vi "Basic_Control_SubVI.vi"(0 "Numeric 2":dbl, 1 "Numeric":dbl, 2 "Numeric 10":dbl, 3 "Numeric 8":dbl, 4 "Numeric 9":dbl, 5 "Numeric 7":dbl, 6 "Numeric 6":dbl, 8 "Numeric 3":dbl, 9 "Tolerance":dbl, 10 "Numeric 4":dbl, 11 "duty cycle (periods) 5":fxp<+,32,0>, 12 "Numeric 5":dbl) -> (16 "Colision?":bool, 18 "duty cycle (periods) 4":fxp<+,32,0>, 19 "Mod1/Drive Direction 2":enum8{"Clockwise", "Counterclockwise"}(ring), 20 "Mod1/Drive Direction 6":enum8{"Clockwise", "Counterclockwise"}(ring), 21 "duty cycle (periods) 3":fxp<+,32,0>, 22 "Mod1/Drive Direction 5":enum8{"Clockwise", "Counterclockwise"}(ring), 23 "duty cycle (periods) 2":fxp<+,32,0>, 24 "Mod1/Drive Direction 4":enum8{"Clockwise", "Counterclockwise"}(ring), 25 "Mod1/Drive Direction 3":enum8{"Clockwise", "Counterclockwise"}(ring), 26 "duty cycle (periods)":fxp<+,32,0>)   [LabVIEW 2014]
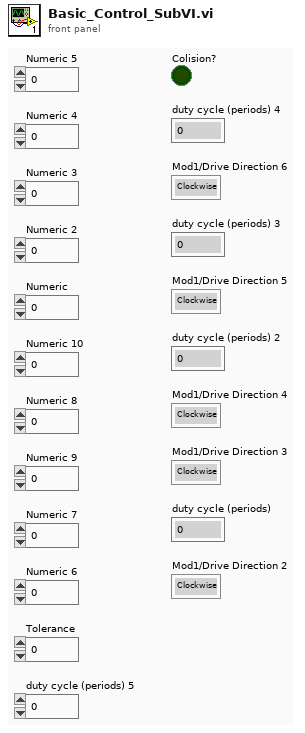
[diagram p1: front panel]
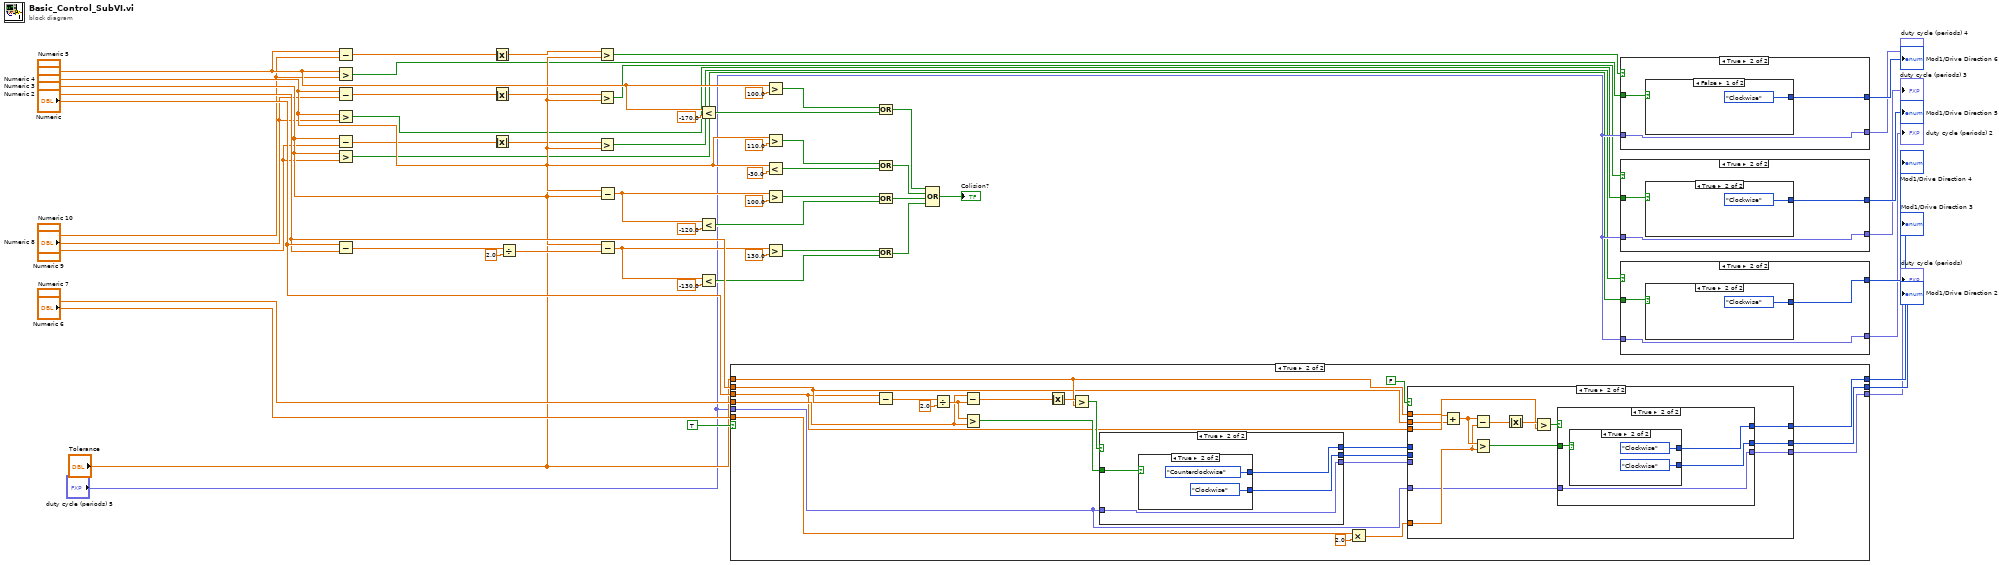
[diagram p0: block diagram]
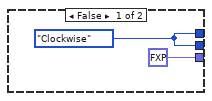
[diagram p2: hidden frame]
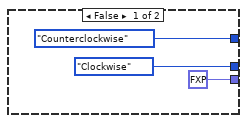
[diagram p4: hidden frame]
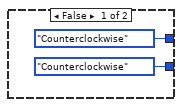
[diagram p5: hidden frame]
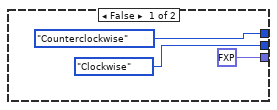
[diagram p6: hidden frame]
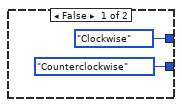
[diagram p7: hidden frame]
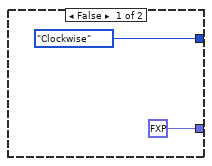
[diagram p8: hidden frame]
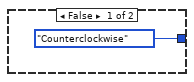
[diagram p9: hidden frame]
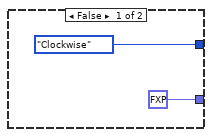
[diagram p10: hidden frame]
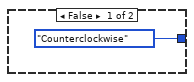
[diagram p11: hidden frame]
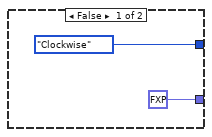
[diagram p12: hidden frame]
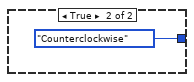
[diagram p13: hidden frame]
diagram:
  n1 = Subtract(x="Numeric 5", y="Numeric 10") -> (x-y=w5:dbl)
  n2 = Greater?(x="Numeric 5", y="Numeric 10") -> (0:w1:bool)
  n3 = Subtract(x="Numeric 4", y="Numeric 8") -> (x-y=w12:dbl)
  n4 = Greater?(x="Numeric 4", y="Numeric 8") -> (0:w2:bool)
  n5 = Subtract(x="Numeric 3", y="Numeric 9") -> (x-y=w9:dbl)
  n6 = Greater?(x="Numeric 3", y="Numeric 9") -> (0:w3:bool)
  n7 = Subtract(x="Numeric", y="Numeric 2") -> (x-y=w49:dbl)
  n8 = Absolute Value(x=w5) -> (abs(x)=w6:dbl)
  n9 = Absolute Value(x=w12) -> (abs(x)=w13:dbl)
  n10 = Absolute Value(x=w9) -> (abs(x)=w10:dbl)
  n11 = Divide(x=w49, y=2.0) -> (x/y=w50:dbl)
  n12 = Greater?(x=w6, y="Tolerance") -> (0:w7:bool)
  n13 = Greater?(x=w13, y="Tolerance") -> (0:w14:bool)
  n14 = Greater?(x=w10, y="Tolerance") -> (0:w15:bool)
  n15 = Subtract(x="Numeric 4", y="Numeric 3") -> (x-y=w29:dbl)
  n16 = Subtract(x="Numeric 3", y=w50) -> (x-y=w34:dbl)
  n17 = Less?(x="Numeric 5", y=-170.0) -> (x < y?=w22:bool)
  n18 = Less?(x=w29, y=-120.0) -> (x < y?=w33:bool)
  n19 = Less?(x=w34, y=-130.0) -> (x < y?=w38:bool)
  n20 = case shown="True" TRUE {
    tunnel: [w61 w84] -> w59
    tunnel: [w61 w83] -> w60
    tunnel: [fxp<+,32,0> 0.0 ("duty cycle (periods)") w82] -> w55
    tunnel: "duty cycle (periods) 5" -> [_ w80]
    tunnel: "Tolerance" -> [_ w73]
    tunnel: "Numeric 2" -> [_ w68]
    tunnel: "Numeric 7" -> [_ w67]
    tunnel: "Numeric" -> [_ w66]
    tunnel: "Numeric 6" -> [_ w65]
    frame False {
      w61 = enum8{"Clockwise", "Counterclockwise"}."Clockwise" ("Mod1/Drive Direction 2")
    }
    frame True {
      n21 = Subtract(x=w66, y=w68) -> (x-y=w72:dbl)
      n22 = Divide(x=w72, y=2.0) -> (x/y=w70:dbl)
      n23 = Subtract(x=w67, y=w70) -> (x-y=w76:dbl)
      n24 = Greater?(x=w70, y=w67) -> (0:w69:bool)
      n25 = Absolute Value(x=w76) -> (abs(x)=w75:dbl)
      n26 = Greater?(x=w75, y=w73) -> (0:w74:bool)
      n27 = case shown="True" w74 {
        tunnel: w80 -> [_ w118]
        tunnel: [fxp<+,32,0> 0.0 ("duty cycle (periods)") w118] -> w79
        tunnel: [enum8{"Clockwise", "Counterclockwise"}."Counterclockwise" ("Mod1/Drive Direction 2") w117] -> w78
        tunnel: [enum8{"Clockwise", "Counterclockwise"}."Clockwise" ("Mod1/Drive Direction 2") w116] -> w77
        tunnel: w69 -> [_ w115]
        frame False {
        }
        frame True {
          n28 = case shown="True" w115 {
            tunnel: [enum8{"Clockwise", "Counterclockwise"}."Clockwise" ("Mod1/Drive Direction 2") enum8{"Clockwise", "Counterclockwise"}."Counterclockwise" ("Mod1/Drive Direction 2")] -> w117
            tunnel: [enum8{"Clockwise", "Counterclockwise"}."Counterclockwise" ("Mod1/Drive Direction 2") enum8{"Clockwise", "Counterclockwise"}."Clockwise" ("Mod1/Drive Direction 2")] -> w116
            frame False {
            }
            frame True {
            }
          }
        }
      }
      n29 = Multiply(x=w65, y=2.0) -> (x*y=w63:dbl)
      n30 = case shown="True" FALSE {
        tunnel: w66 -> [_ w100]
        tunnel: w68 -> [_ w99]
        tunnel: w63 -> [_ w95]
        tunnel: w73 -> [_ w93]
        tunnel: [w86 w91] -> w84
        tunnel: [w85 w90] -> w83
        tunnel: w80 -> [_ w89]
        tunnel: [w87 w88] -> w82
        tunnel: w79 -> [w87 _]
        tunnel: w78 -> [w86 _]
        tunnel: w77 -> [w85 _]
        frame False {
        }
        frame True {
          n31 = Add(x=w100, y=w99) -> (x+y=w96:dbl)
          n32 = Subtract(x=w96, y=w95) -> (x-y=w97:dbl)
          n33 = Greater?(x=w96, y=w95) -> (0:w98:bool)
          n34 = Absolute Value(x=w97) -> (abs(x)=w94:dbl)
          n35 = Greater?(x=w94, y=w93) -> (0:w92:bool)
          n36 = case shown="True" w92 {
            tunnel: w98 -> [_ w106]
            tunnel: [fxp<+,32,0> 0.0 ("duty cycle (periods)") w107] -> w88
            tunnel: [enum8{"Clockwise", "Counterclockwise"}."Counterclockwise" ("Mod1/Drive Direction 2") w105] -> w91
            tunnel: [enum8{"Clockwise", "Counterclockwise"}."Clockwise" ("Mod1/Drive Direction 2") w104] -> w90
            tunnel: w89 -> [_ w107]
            frame False {
            }
            frame True {
              n37 = case shown="True" w106 {
                tunnel: [enum8{"Clockwise", "Counterclockwise"}."Counterclockwise" ("Mod1/Drive Direction 2") enum8{"Clockwise", "Counterclockwise"}."Clockwise" ("Mod1/Drive Direction 2")] -> w105
                tunnel: [enum8{"Clockwise", "Counterclockwise"}."Counterclockwise" ("Mod1/Drive Direction 2") enum8{"Clockwise", "Counterclockwise"}."Clockwise" ("Mod1/Drive Direction 2")] -> w104
                frame False {
                }
                frame True {
                }
              }
            }
          }
        }
      }
    }
  }
  "Mod1/Drive Direction 2" <- w60
  "Mod1/Drive Direction 3" <- w59
  "duty cycle (periods)" <- w55
  n38 = Greater?(x="Numeric 5", y=100.0) -> (0:w21:bool)
  n39 = Greater?(x="Numeric 4", y=110.0) -> (0:w25:bool)
  n40 = Less?(x="Numeric 4", y=-30.0) -> (x < y?=w26:bool)
  n41 = Greater?(x=w29, y=100.0) -> (0:w32:bool)
  n42 = Greater?(x=w34, y=130.0) -> (0:w37:bool)
  n43 = Or(x=w21, y=w22) -> (x .or. y?=w39:bool)
  n44 = Or(x=w25, y=w26) -> (x .or. y?=w40:bool)
  n45 = Or(x=w32, y=w33) -> (x .or. y?=w41:bool)
  n46 = Or(x=w37, y=w38) -> (x .or. y?=w42:bool)
  n47 = Compound Arithmetic op=OR(w39, w40, w41, w42) -> (→"Colision?":bool)
  n48 = case shown="True" w7 {
    tunnel: w1 -> [_ w127]
    tunnel: "duty cycle (periods) 5" -> [_ w125]
    tunnel: [enum8{"Clockwise", "Counterclockwise"}."Clockwise" ("Mod1/Drive Direction 2") w126] -> w56
    tunnel: [fxp<+,32,0> 0.0 ("duty cycle (periods)") w125] -> w52
    frame False {
    }
    frame True {
      n49 = case shown="False" w127 {
        tunnel: [enum8{"Clockwise", "Counterclockwise"}."Clockwise" ("Mod1/Drive Direction 2") enum8{"Clockwise", "Counterclockwise"}."Counterclockwise" ("Mod1/Drive Direction 2")] -> w126
        frame False {
        }
        frame True {
        }
      }
    }
  }
  "Mod1/Drive Direction 6" <- w56
  "duty cycle (periods) 4" <- w52
  n50 = case shown="True" w14 {
    tunnel: w2 -> [_ w134]
    tunnel: "duty cycle (periods) 5" -> [_ w132]
    tunnel: [enum8{"Clockwise", "Counterclockwise"}."Clockwise" ("Mod1/Drive Direction 2") w133] -> w57
    tunnel: [fxp<+,32,0> 0.0 ("duty cycle (periods)") w132] -> w53
    frame False {
    }
    frame True {
      n51 = case shown="True" w134 {
        tunnel: [enum8{"Clockwise", "Counterclockwise"}."Counterclockwise" ("Mod1/Drive Direction 2") enum8{"Clockwise", "Counterclockwise"}."Clockwise" ("Mod1/Drive Direction 2")] -> w133
        frame False {
        }
        frame True {
        }
      }
    }
  }
  "Mod1/Drive Direction 5" <- w57
  "duty cycle (periods) 3" <- w53
  n52 = case shown="True" w15 {
    tunnel: w3 -> [_ w141]
    tunnel: "duty cycle (periods) 5" -> [_ w139]
    tunnel: [enum8{"Clockwise", "Counterclockwise"}."Clockwise" ("Mod1/Drive Direction 2") w140] -> w58
    tunnel: [fxp<+,32,0> 0.0 ("duty cycle (periods)") w139] -> w54
    frame False {
    }
    frame True {
      n53 = case shown="True" w141 {
        tunnel: [enum8{"Clockwise", "Counterclockwise"}."Counterclockwise" ("Mod1/Drive Direction 2") enum8{"Clockwise", "Counterclockwise"}."Clockwise" ("Mod1/Drive Direction 2")] -> w140
        frame False {
        }
        frame True {
        }
      }
    }
  }
  "Mod1/Drive Direction 4" <- w58
  "duty cycle (periods) 2" <- w54
